vi "test Parse Bitfile EST Clusters Version.vi"(8 "error in (no error)":errorcluster, 11 "TestCase in":refnum<class "Bitfile Parsing Test Case.lvclass">) -> (0 "error out":errorcluster, 3 "TestCase out":refnum<class "Bitfile Parsing Test Case.lvclass">)   [LabVIEW 2017, in "Bitfile Parsing Test Case.lvclass"]
uses:
  Bitfile Parsing Test Case.lvclass
  Shared/Bitfile EST Version.ctl
  <userlib>/_OpenG.lib/file/file.llb/Append Path to Root if Relative - Scalar__ogtk.vi
  <vilib>/addons/_JKI Toolkits/VI Tester/TestCase.llb/TestCase.lvclass
  Shared/Engine Simulation Toolkit Shared.lvlib
  System Explorer/Engine Simulation Toolkit System Explorer.lvlib
  C:/Program Files (x86)/National Instruments/LabVIEW 2017/vi.lib/addons/_JKI Toolkits/VI Tester/TestCase.llb/TestCase.lvclass
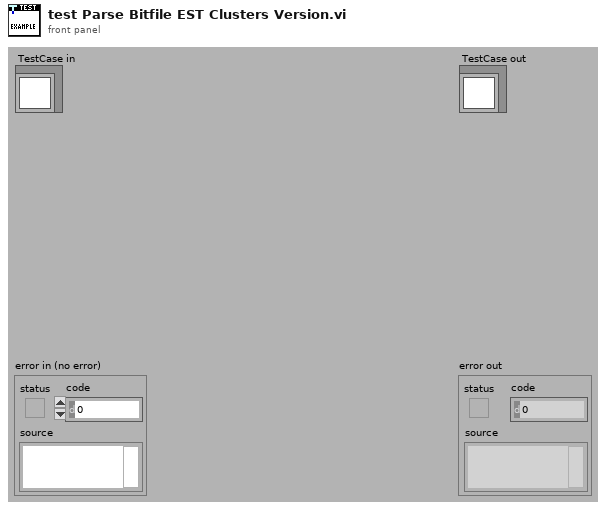
[diagram p1: front panel]
types:
  T1 = typedef "Engine Simulation Toolkit Shared.lvlib/Bitfile EST Version.ctl" = enum16{"1.0", "1.1", "1.2", "1.3", "1.4"}
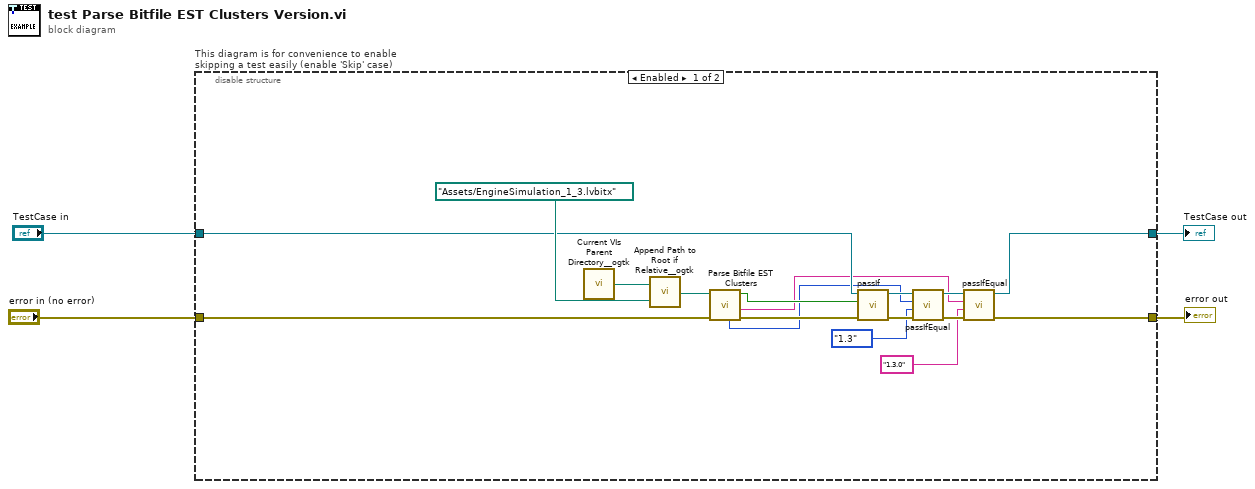
[diagram p0: block diagram]
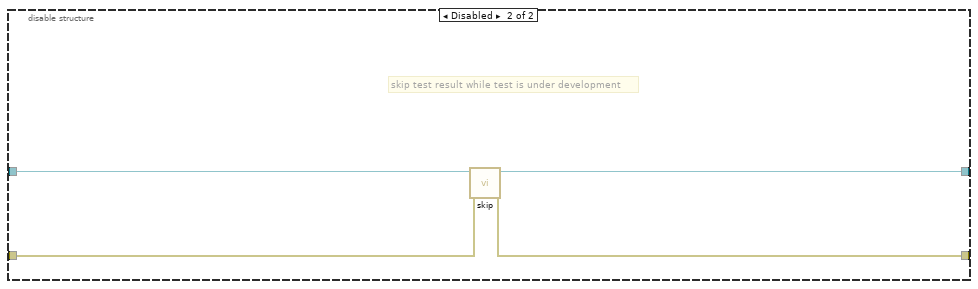
[diagram p2: hidden frame]
diagram:
  n1 = disable-structure "This diagram is for convenience to enable skipping a test easily (enable 'Skip' case)" shown="Enabled" {
    disable-tunnel: "TestCase in" -> [w19 w25]
    disable-tunnel: [w13 w23] -> w1
    disable-tunnel: [w16 w24] -> w3
    disable-tunnel: "error in (no error)" -> [w10 w22]
    frame Enabled {
      n2 = call <userlib>:"Current VIs Parent Directory__ogtk.vi"() -> ("Parent Directory (+ Relative)"=w21:path)  [unwired: 5 in]
      n3 = call-poly <userlib>:"Append Path to Root if Relative__ogtk.vi"("Absolute or Relative Path"=path "Assets/EngineSimulation_1_3.lvbitx" ("bitfile path"), "Root Path"=w21) -> ("Absolute or Appended Path"=w5:path)
      n4 = call "Parse Bitfile EST Clusters.vi"("error in (no error)"=w10, "bitfile path"=w5) -> ("error out"=w9:errorcluster, "version"=w6:string, "valid bitfile"=w8:bool, "EST version enum"=w7:T1)  [unwired: 5 in, 1 out]
      n5 = call-dynamic "passIf.vi"("error in (no error)"=w9, "pass"=w8, "TestCase in"=w19) -> ("error out"=w18:errorcluster, "TestCase out"=w14:refnum<class "Bitfile Parsing Test Case.lvclass">)  [unwired: 7 in]
      n6 = call-dynamic "passIfEqual.vi"("error in (no error)"=w18, "y"=Bitfile_EST_Version."1.3" ("EST version enum"), "x"=w7, "TestCase in"=w14) -> ("error out"=w17:errorcluster, "TestCase out"=w15:refnum<class "Bitfile Parsing Test Case.lvclass">)  [unwired: 6 in]
      n7 = call-dynamic "passIfEqual.vi"("error in (no error)"=w17, "y"="1.3.0" ("EST version string"), "x"=w6, "TestCase in"=w15) -> ("error out"=w16:errorcluster, "TestCase out"=w13:refnum<class "Bitfile Parsing Test Case.lvclass">)  [unwired: 6 in]
    }
    frame Disabled {
      # "skip test result while test is under development"
      n8 = call <vilib>:"skip.vi"("error in (no error)"=w22, "TestCase in"=w25) -> ("error out"=w24:errorcluster, "TestCase out"=w23:refnum<class "Bitfile Parsing Test Case.lvclass">)  [unwired: 8 in]
    }
  }
  "error out" <- w3
  "TestCase out" <- w1
